vi "TimeRecToTimeInt.vi"(1 "TimeRec":T1) -> (0 "timeInt":u32)   [LabVIEW 2009]
uses:
  TimeRec.ctl
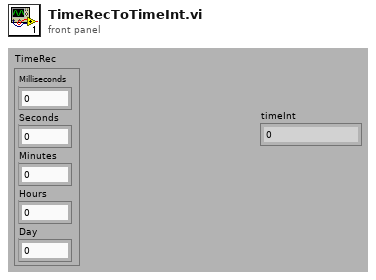
[diagram p1: front panel]
types:
  T1 = typedef "TimeRec.ctl" = cluster{"Milliseconds":u32, "Seconds":u32, "Minutes":u32, "Hours":u32, "Day":u32}
  T2 = cluster{"Boolean array[0]":bool, "Boolean array[1]":bool, "Boolean array[2]":bool, "Boolean array[3]":bool, "Boolean array[4]":bool, "Boolean array[5]":bool, "Boolean array[6]":bool, "Boolean array[7]":bool, "Boolean array[8]":bool, "Boolean array[9]":bool}
  T3 = cluster{"Boolean array[0]":bool, "Boolean array[1]":bool, "Boolean array[2]":bool, "Boolean array[3]":bool, "Boolean array[4]":bool, "Boolean array[5]":bool}
  T4 = cluster{"Boolean array[0]":bool, "Boolean array[1]":bool, "Boolean array[2]":bool, "Boolean array[3]":bool, "Boolean array[4]":bool}
  T5 = cluster{"Boolean array[0]":bool, "Boolean array[1]":bool, "Boolean array[2]":bool, "Boolean array[3]":bool, "Boolean array[4]":bool, "Boolean array[5]":bool, "Boolean array[6]":bool, "Boolean array[7]":bool, "Boolean array[8]":bool, "Boolean array[9]":bool, "Boolean array[0]":bool, "Boolean array[1]":bool, "Boolean array[2]":bool, "Boolean array[3]":bool, "Boolean array[4]":bool, "Boolean array[5]":bool, "Boolean array[0]":bool, "Boolean array[1]":bool, "Boolean array[2]":bool, "Boolean array[3]":bool, "Boolean array[4]":bool, "Boolean array[5]":bool, "Boolean array[0]":bool, "Boolean array[1]":bool, "Boolean array[2]":bool, "Boolean array[3]":bool, "Boolean array[4]":bool, "Boolean array[0]":bool, "Boolean array[1]":bool, "Boolean array[2]":bool, "Boolean array[3]":bool, "Boolean array[4]":bool}
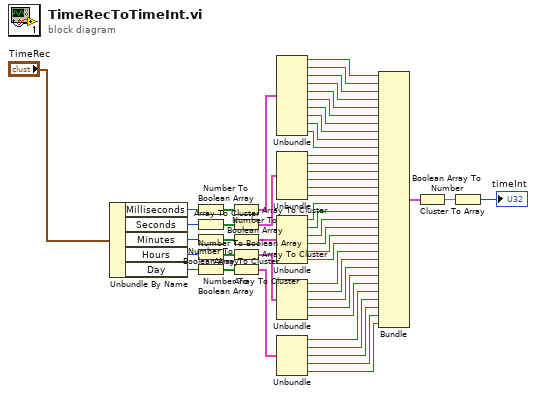
[diagram p0: block diagram]
diagram:
  n1 = Unbundle By Name("TimeRec") -> ("Milliseconds"=w13:u32, "Seconds"=w12:u32, "Minutes"=w11:u32, "Hours"=w10:u32, "Day"=w6:u32)
  n2 = Number To Boolean Array(number=w13) -> (Boolean array=w17:bool[])
  n3 = Number To Boolean Array(number=w12) -> (Boolean array=w16:bool[])
  n4 = Number To Boolean Array(number=w11) -> (Boolean array=w15:bool[])
  n5 = Number To Boolean Array(number=w10) -> (Boolean array=w14:bool[])
  n6 = Number To Boolean Array(number=w6) -> (Boolean array=w7:bool[])
  n7 = Array To Cluster(array=w17) -> (cluster=w18:T2)
  n8 = Array To Cluster(array=w16) -> (cluster=w30:T3)
  n9 = Array To Cluster(array=w15) -> (cluster=w29:T3)
  n10 = Array To Cluster(array=w14) -> (cluster=w43:T4)
  n11 = Array To Cluster(array=w7) -> (cluster=w9:T4)
  n12 = Unbundle(w18) -> ("Boolean array[0]"=w19:bool, "Boolean array[1]"=w20:bool, "Boolean array[2]"=w21:bool, "Boolean array[3]"=w22:bool, "Boolean array[4]"=w23:bool, "Boolean array[5]"=w24:bool, "Boolean array[6]"=w25:bool, "Boolean array[7]"=w26:bool, "Boolean array[8]"=w27:bool, "Boolean array[9]"=w28:bool)
  n13 = Unbundle(w30) -> ("Boolean array[0]"=w31:bool, "Boolean array[1]"=w32:bool, "Boolean array[2]"=w33:bool, "Boolean array[3]"=w34:bool, "Boolean array[4]"=w35:bool, "Boolean array[5]"=w36:bool)
  n14 = Unbundle(w29) -> ("Boolean array[0]"=w37:bool, "Boolean array[1]"=w38:bool, "Boolean array[2]"=w39:bool, "Boolean array[3]"=w40:bool, "Boolean array[4]"=w41:bool, "Boolean array[5]"=w42:bool)
  n15 = Unbundle(w43) -> ("Boolean array[0]"=w44:bool, "Boolean array[1]"=w45:bool, "Boolean array[2]"=w46:bool, "Boolean array[3]"=w47:bool, "Boolean array[4]"=w48:bool)
  n16 = Unbundle(w9) -> ("Boolean array[0]"=w8:bool, "Boolean array[1]"=w5:bool, "Boolean array[2]"=w4:bool, "Boolean array[3]"=w3:bool, "Boolean array[4]"=w2:bool)
  n17 = Bundle("Boolean array[0]"=w19, "Boolean array[1]"=w20, "Boolean array[2]"=w21, "Boolean array[3]"=w22, "Boolean array[4]"=w23, "Boolean array[5]"=w24, "Boolean array[6]"=w25, "Boolean array[7]"=w26, "Boolean array[8]"=w27, "Boolean array[9]"=w28, "Boolean array[0]"=w31, "Boolean array[1]"=w32, "Boolean array[2]"=w33, "Boolean array[3]"=w34, "Boolean array[4]"=w35, "Boolean array[5]"=w36, "Boolean array[0]"=w37, "Boolean array[1]"=w38, "Boolean array[2]"=w39, "Boolean array[3]"=w40, "Boolean array[4]"=w41, "Boolean array[5]"=w42, "Boolean array[0]"=w44, "Boolean array[1]"=w45, "Boolean array[2]"=w46, "Boolean array[3]"=w47, "Boolean array[4]"=w48, "Boolean array[0]"=w8, "Boolean array[1]"=w5, "Boolean array[2]"=w4, "Boolean array[3]"=w3, "Boolean array[4]"=w2) -> (w49:T5)  [unwired: 1 in]
  n18 = Cluster To Array(cluster=w49) -> (array=w50:bool[])
  n19 = Boolean Array To Number(Boolean array=w50) -> (number=→"timeInt":u32)
